vi "校验用户信息.vi"(1 "密码":string, 2 "用户名":string) -> (0 "布尔":bool)   [LabVIEW 2013]
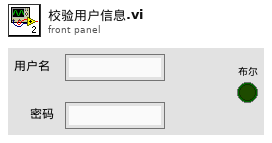
[diagram p1: front panel]
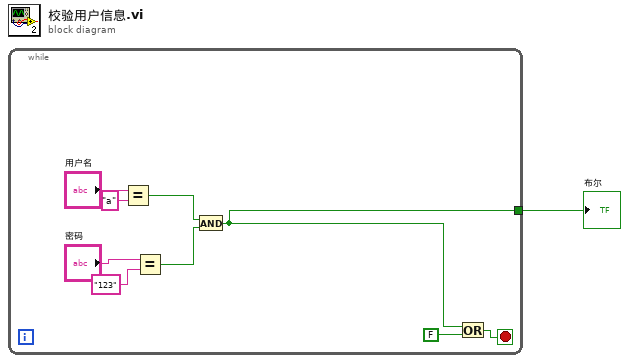
[diagram p0: block diagram]
diagram:
  n1 = while {
    tunnel: [w2] -> w1
    stop <- w8 stop-if-true
    n2 = Equal?(x="用户名", y="a") -> (x = y?=w4:bool)
    n3 = Equal?(x="密码", y="123") -> (x = y?=w3:bool)
    n4 = And(x=w4, y=w3) -> (x .and. y?=w2:bool)
    n5 = Or(x=w2, y=FALSE) -> (x .or. y?=w8:bool)
  }
  "布尔" <- w1
